vi "Actor.vi"(4 "Debug Alias":string, 6 "Open Actor Core front panel? (F)":bool, 7 "error feedback":refnum<queue>, 9 "Actor":refnum<class "Actor.lvclass">, 10 "queue of queues":refnum<queue>, 11 "Message Enqueuer":refnum<class "Message Enqueuer.lvclass">) -> ()   [LabVIEW 2017, in "Actor Framework.lvlib" / "Actor.lvclass"]
doc: "(<B>Filename</B>: Actor Framework.lvlib:Actor.lvclass:Actor.vi)\n\nActor.vi is the top-level VI that is launched to be the functional aspect of the actor object. It is a wrapper around Actor Core.vi, which is where the actor defines most of its specific behavior. Actor.vi takes care of creating the caller-to-actor queue and brokering the exchange of enqueuers with the caller. It also handles all the cleanup when Actor Core.vi completes. It is not dynamic dispatch -- users of the actor framework generally don't need to understand what's being done in this function."
uses:
  <vilib>/ActorFramework/Actor/Actor.lvclass
  <vilib>/ActorFramework/Message Enqueuer/Message Enqueuer.lvclass
  <vilib>/ActorFramework/Message Enqueuer/Message Enqueuer.lvclass/Message Enqueuer.ctl
  <vilib>/ActorFramework/Actor/Actor.lvclass/Actor.ctl
  <vilib>/ActorFramework/LastAck/Last Ack.lvclass/Last Ack.ctl
  <vilib>/ActorFramework/Message Enqueuer/Enqueue Critical.vi
  <vilib>/ActorFramework/LastAck/Last Ack.lvclass
  e:/builds/penguin/labview/branches/2017/dev/dist/vi.lib/ActorFramework/Message/Message.lvclass
  <vilib>/ActorFramework/Message Priority Queue/Priority Enqueue.vi
  <vilib>/ActorFramework/Message/Message.lvclass
  <vilib>/ActorFramework/Message Priority Queue/Message Priority Queue.lvclass
  <resource>/AFDebug/AF Debug.lvlib
panel:
  out "error out":errorcluster
  # "The error out is here only as an aid to debugging if necessary."
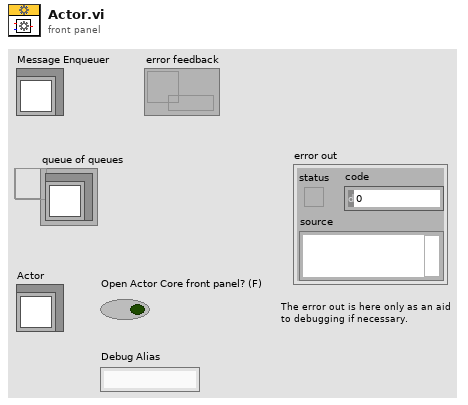
[diagram p1: front panel]
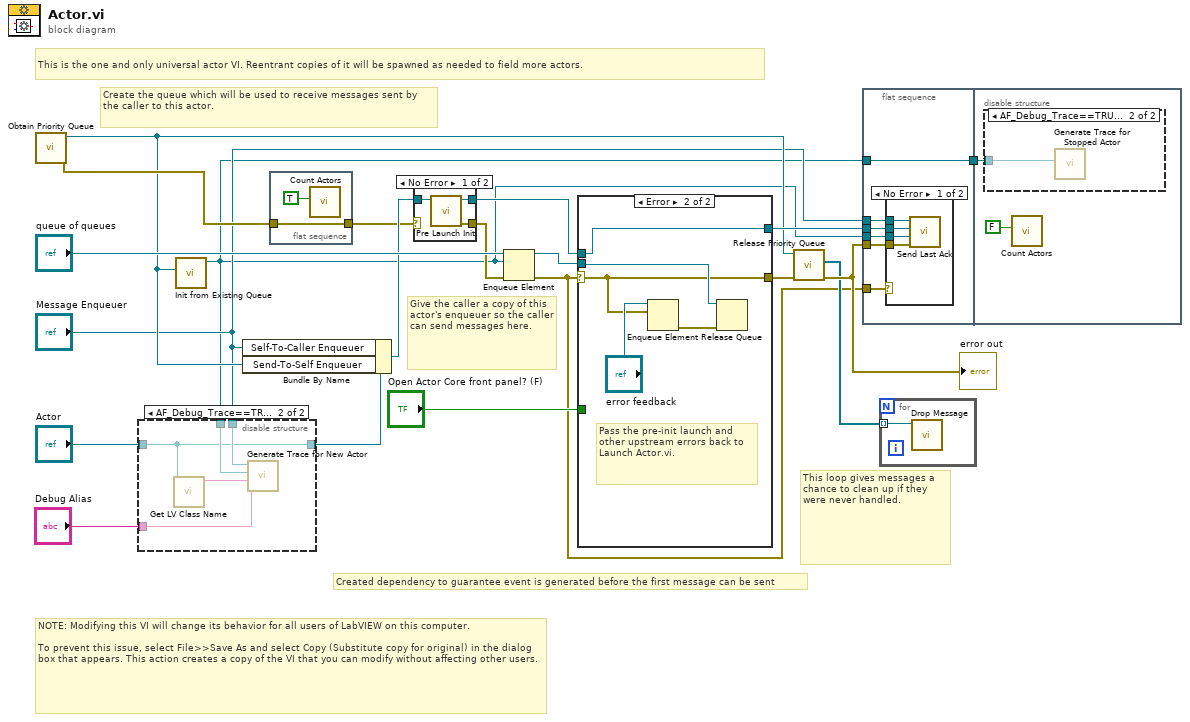
[diagram p0: block diagram]
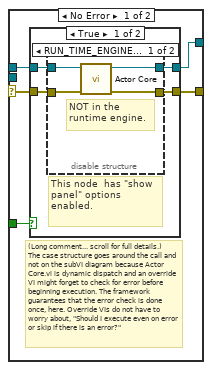
[diagram p6: hidden frame]
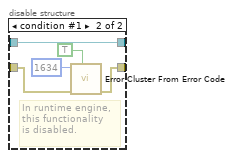
[diagram p7: hidden frame]
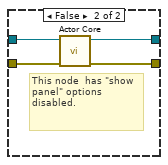
[diagram p8: hidden frame]
diagram:
  # "Created dependency to guarantee event is generated before the first message can be sent"
  # "NOTE: Modifying this VI will change its behavior for all users of LabVIEW on this computer.\n\nTo prevent this issue, select File>>Save As and select Copy (Substitute copy for original) in the dialog box that appears. This action creates a copy of the VI that you can modify without affecting other users."
  # "This loop gives messages a chance to clean up if they were never handled."
  # "Give the caller a copy of this actor's enqueuer so the caller can send messages here."
  # "Create the queue which will be used to receive messages sent by the caller to this actor."
  # "This is the one and only universal actor VI. Reentrant copies of it will be spawned as needed to field more actors."
  n1 = call <vilib>:"Obtain Priority Queue.vi"() -> ("error out"=w9:errorcluster, "Priority Queue"=w8:refnum<class "Message Priority Queue.lvclass">)  [unwired: 10 in]
  n2 = call <vilib>:"Init from Existing Queue.vi"("Priority Queue"=w8) -> ("Message Enqueuer"=w2:refnum<class "Message Enqueuer.lvclass">)  [unwired: 10 in]
  n3 = disable-structure shown="AF_Debug_Trace==TRUE" {
    disable-tunnel: "Actor" -> [w21 w22]
    disable-tunnel: "Message Enqueuer" -> [_ w26]
    disable-tunnel: w2 -> [_ w25]
    disable-tunnel: "Debug Alias" -> [_ w23]
    disable-tunnel: [w21 w22] -> w5
    frame condition #0 (active) {
    }
    frame condition #1 {
      n4 = call <vilib>:"Get LV Class Name.vi"("object"=w22) -> ("class name"=w24:string)  [unwired: 9 in, 1 out]
      n5 = call <resource>:"Generate Trace for New Actor.vi"("Debug Alias"=w23, "Class Name"=w24, "Actor Enqueuer"=w25, "Caller Enqueuer"=w26) -> ()  [unwired: 8 in]
    }
  }
  n6 = Bundle By Name(cluster=w5, "Self-To-Caller Enqueuer"="Message Enqueuer", "Send-To-Self Enqueuer"=w8) -> (w15:refnum<class "Actor.lvclass">)
  n7 = flat-sequence {
    tunnel: [w27] -> w10
    tunnel: w9 -> [w27]
    frame #0 {
      n8 = call <vilib>:"Count Actors.vi"("Increment?"=TRUE) -> ()  [unwired: 11 in]
    }
  }
  n9 = case shown="No Error" w10 {
    selector: w10 -> [_ w33]
    tunnel: w15 -> [w31 w32]
    tunnel: [w30 w32] -> w14
    tunnel: [w29 w33] -> w11
    frame No Error {
      n10 = call-dynamic "Pre Launch Init.vi"("Actor in"=w31) -> ("error out"=w29:errorcluster, "Actor out"=w30:refnum<class "Actor.lvclass">)  [unwired: 9 in]
    }
    frame Error {
    }
  }
  n11 = Enqueue Element(queue="queue of queues", element=w2, error in (no error)=w11) -> (queue out=w13:refnum<queue>, error out=w1:errorcluster)  [unwired: 1 in, 1 out]
  n12 = case shown="Error" w1 {
    selector: w1 -> [w35 w56]
    tunnel: w14 -> [w36 w60]
    tunnel: [w38 w56] -> w20
    tunnel: [w37 w60] -> w18
    tunnel: w13 -> [_ w59]
    tunnel: "Open Actor Core front panel? (F)" -> [w34 _]
    frame No Error {
      # "(Long comment... scroll for full details.)\nThe case structure goes around the call and not on the subVI diagram because Actor Core.vi is dynamic dispatch and an override VI might forget to check for error before beginning execution. The framework guarantees that the error check is done once, here. Override VIs do not have to worry about, \"Should I execute even on error or skip if there is an error?\""
      n13 = case shown="True" w34 {
        tunnel: [w42 w55] -> w38
        tunnel: [w41 w54] -> w37
        tunnel: w36 -> [w40 w53]
        tunnel: w35 -> [w39 w52]
        frame True {
          # "This node  has \"show panel\" options enabled."
          n14 = disable-structure shown="RUN_TIME_ENGINE==False" {
            disable-tunnel: [w46 w50] -> w42
            disable-tunnel: [w45 w51] -> w41
            disable-tunnel: w40 -> [w44 w51]
            disable-tunnel: w39 -> [w43 w49]
            frame condition #0 (active) {
              # "NOT in the \nruntime engine."
              n15 = call-dynamic "Actor Core.vi"("error in"=w43, "Actor in"=w44) -> ("error out"=w46:errorcluster, "Actor out"=w45:refnum<class "Actor.lvclass">)  [unwired: 8 in]
            }
            frame condition #1 {
              # "In runtime engine,\nthis functionality\nis disabled."
              n16 = call <vilib>:"Error Cluster From Error Code.vi"("show call chain? (False)"=TRUE, "error in (no error)"=w49, "error code (0)"=1634) -> ("error out"=w50:errorcluster)  [unwired: 6 in]
            }
          }
        }
        frame False {
          # "This node  has \"show panel\" options disabled."
          n17 = call-dynamic "Actor Core.vi"("error in"=w52, "Actor in"=w53) -> ("error out"=w55:errorcluster, "Actor out"=w54:refnum<class "Actor.lvclass">)  [unwired: 8 in]
        }
      }
    }
    frame Error {
      # "Pass the pre-init launch and other upstream errors back to Launch Actor.vi."
      n18 = Enqueue Element(queue="error feedback", element=w56) -> (error out=w57:errorcluster)  [unwired: 2 in, 2 out]
      n19 = Release Queue(queue=w59, error in (no error)=w57) -> ()  [unwired: 1 in, 3 out]
    }
  }
  n20 = call <vilib>:"Release Priority Queue.vi"("error in (no error)"=w20, "Priority Queue"=w8) -> ("error out"=w19:errorcluster, "remaining elements"=w16:refnum<class "Message.lvclass">[])  [unwired: 8 in]
  "error out" <- w19
  n21 = flat-sequence {
    tunnel: w19 -> [w66]
    tunnel: w18 -> [w65]
    tunnel: "Message Enqueuer" -> [w64]
    tunnel: w2 -> [w63]
    tunnel: [w62] -> w4
    tunnel: w2 -> [w62]
    tunnel: w1 -> [w61]
    tunnel: w4 -> [w71]
    frame #0 {
      n22 = case shown="No Error" w61 {
        tunnel: w66 -> [w70 _]
        tunnel: w65 -> [w69 _]
        tunnel: w64 -> [w68 _]
        tunnel: w63 -> [w67 _]
        frame No Error {
          n23 = call <vilib>:"Send Last Ack.vi"("error from actor"=w70, "Caller-to-Actor Enqueuer"=w67, "Actor"=w69, "Message Enqueuer"=w68) -> ()  [unwired: 8 in]
        }
        frame Error {
        }
      }
    }
    frame #1 {
      n24 = disable-structure shown="AF_Debug_Trace==TRUE" {
        disable-tunnel: w71 -> [_ w73]
        frame condition #0 (active) {
        }
        frame condition #1 {
          n25 = call <resource>:"Generate Trace for Stopped Actor.vi"("Actor Enqueuer"=w73) -> ()  [unwired: 11 in]
        }
      }
      n26 = call <vilib>:"Count Actors.vi"("Increment?"=FALSE) -> ()  [unwired: 11 in]
    }
  }
  n27 = for {
    tunnel: w16 -> [w74] mode=indexing
    n28 = call <vilib>:"Drop Message.vi"("Message in"=w74) -> ()  [unwired: 11 in]
  }
